vi "Peak Detection.vi"(7 "error in (no error)":errorcluster, 10 "Graph Data In":T1) -> (0 "error out":errorcluster, 2 "New Graph Data Out":T1)   [LabVIEW 2013, in "Diode Characterization.lvlib" / "Diode IV.lvclass"]
doc: "Detects up to 10 peaks per waveform that are above the threshold determined by the cursor on the graph. Output is in the form of an array of annotations that can be displayed on the graph alongside the input waveforms."
uses:
  Diode IV.lvclass
  graphdata.ctl
  <vilib>/Utility/miscctls.llb/LVAnnotationListTypeDef.ctl
  <vilib>/Utility/miscctls.llb/LVCursorListTypeDef.ctl
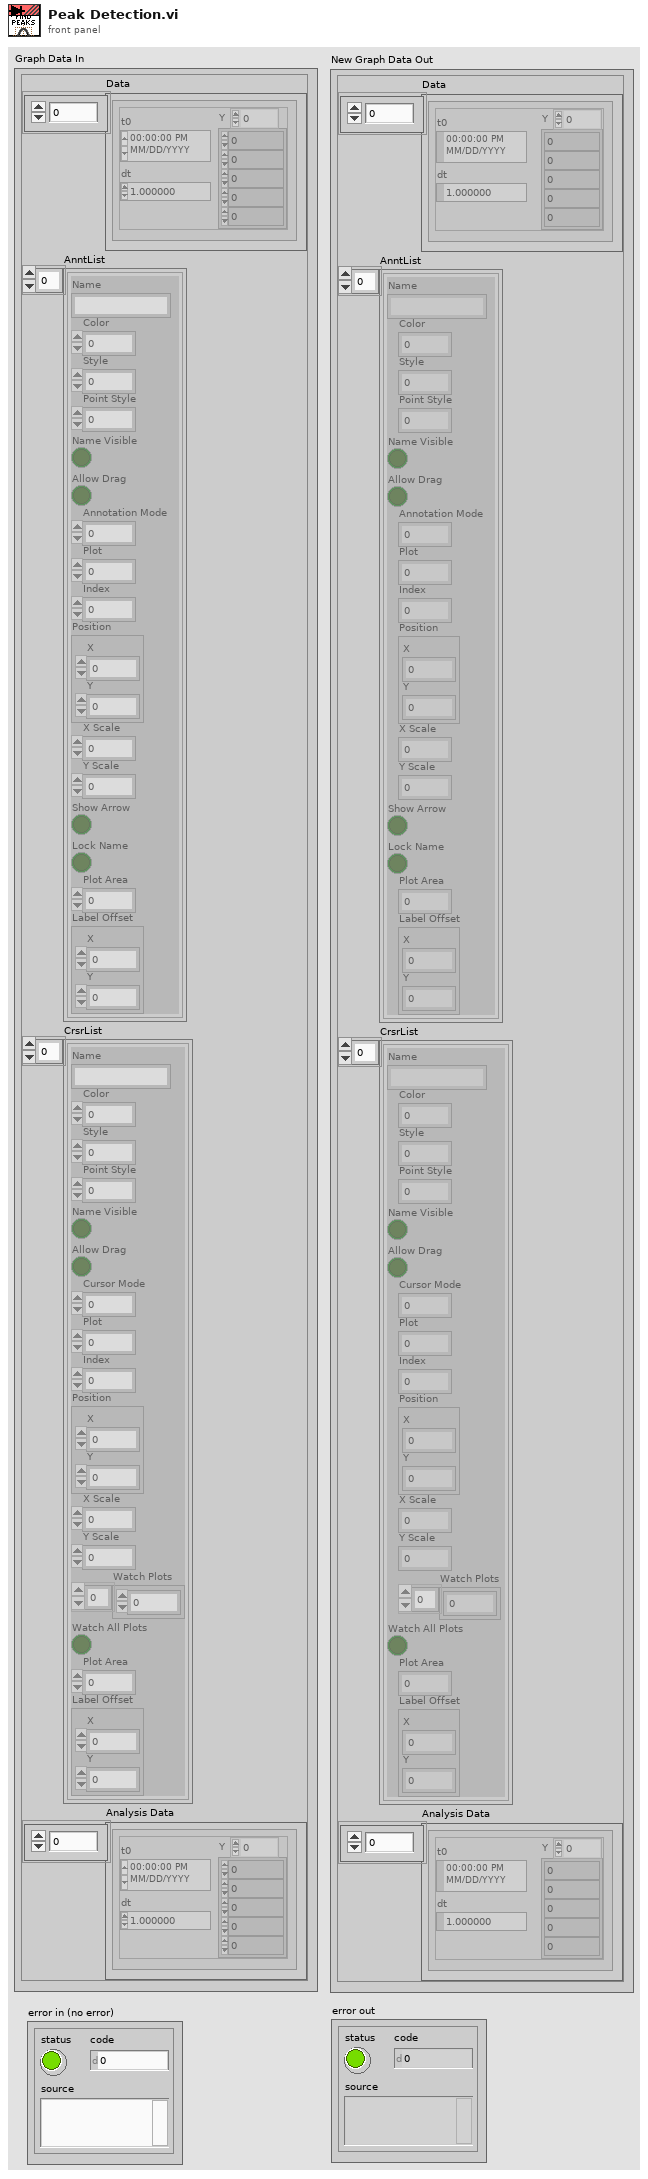
[diagram p1: front panel]
types:
  T1 = typedef "Diode Characterization.lvlib/Diode IV.lvclass/graphdata.ctl" = cluster{"Data":waveform(dbl)[], "AnntList":T2, "CrsrList":T3, "Analysis Data":waveform(dbl)[]}
  T2 = typedef "LVAnnotationListTypeDef.ctl" = cluster{"Name":string, "Color":u32, "Style":u8, "Point Style":u8, "Name Visible":bool, "Allow Drag":bool, "Annotation Mode":u32, "Plot":i32, "Index":i32, "Position":cluster{"X":dbl, "Y":dbl}, "X Scale":u32, "Y Scale":u32, "Show Arrow":bool, "Lock Name":bool, "Plot Area":i32, "Label Offset":cluster{"X":dbl, "Y":dbl}}[]
  T3 = typedef "LVCursorListTypeDef.ctl" = cluster{"Name":string, "Color":u32, "Style":u8, "Point Style":u8, "Name Visible":bool, "Allow Drag":bool, "Cursor Mode":u32, "Plot":i32, "Index":i32, "Position":cluster{"X":dbl, "Y":dbl}, "X Scale":u32, "Y Scale":u32, "Watch Plots":i32[], "Watch All Plots":bool, "Plot Area":i32, "Label Offset":cluster{"X":dbl, "Y":dbl}}[]
  T4 = cluster{"Name":string, "Color":u32, "Style":u8, "Point Style":u8, "Name Visible":bool, "Allow Drag":bool, "Cursor Mode":u32, "Plot":i32, "Index":i32, "Position":cluster{"X":dbl, "Y":dbl}, "X Scale":u32, "Y Scale":u32, "Watch Plots":i32[], "Watch All Plots":bool, "Plot Area":i32, "Label Offset":cluster{"X":dbl, "Y":dbl}}
  T5 = cluster{"Name":string, "Color":u32, "Style":u8, "Point Style":u8, "Name Visible":bool, "Allow Drag":bool, "Annotation Mode":u32, "Plot":i32, "Index":i32, "Position":cluster{"X":dbl, "Y":dbl}, "X Scale":u32, "Y Scale":u32, "Show Arrow":bool, "Lock Name":bool, "Plot Area":i32, "Label Offset":cluster{"X":dbl, "Y":dbl}}[]
  T6 = cluster{"Name":string, "Color":u32, "Style":u8, "Point Style":u8, "Name Visible":bool, "Allow Drag":bool, "Annotation Mode":u32, "Plot":i32, "Index":i32, "Position":cluster{"X":dbl, "Y":dbl}, "X Scale":u32, "Y Scale":u32, "Show Arrow":bool, "Lock Name":bool, "Plot Area":i32, "Label Offset":cluster{"X":dbl, "Y":dbl}}
  T7 = cluster{"Name":string, "Color":u32, "Style":u8, "Point Style":u8, "Name Visible":bool, "Allow Drag":bool, "Cursor Mode":u32, "Plot":i32, "Index":i32, "Position":cluster{"X":dbl, "Y":dbl}, "X Scale":u32, "Y Scale":u32, "Watch Plots":i32[], "Watch All Plots":bool, "Plot Area":i32, "Label Offset":cluster{"X":dbl, "Y":dbl}}[]
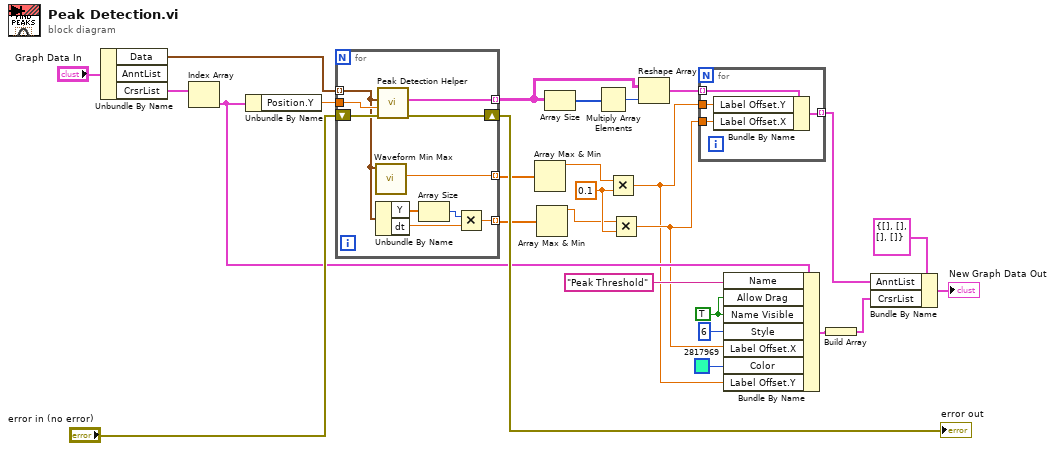
[diagram p0: block diagram]
diagram:
  w6 = 0.1 ("y")
  w14 = TRUE ("Allow Drag")
  n1 = Unbundle By Name("Graph Data In") -> ("Data"=w23:waveform(dbl)[], "CrsrList"=w24:T3)  [unwired: 1 out]
  n2 = Index Array(array=w24) -> (element=w17:T4)  [unwired: 1 in]
  n3 = Unbundle By Name(w17) -> ("Position.Y"=w18:dbl)
  n4 = for {
    tunnel: w23 -> [w29] mode=indexing
    tunnel: [w37] -> w21 mode=indexing
    tunnel: w18 -> [w36]
    shift-right: [w34] -> w27
    shift-left: "error in (no error)" -> [w35]
    tunnel: [w33] -> w9 mode=indexing
    tunnel: [w28] -> w8 mode=indexing
    n5 = call <vilib>:"Waveform Min Max.vi"("waveform in"=w29) -> ("Y max"=w33:dbl)  [unwired: 5 in, 5 out]
    n6 = Unbundle By Name(w29) -> ("Y"=w30:dbl[], "dt"=w32:dbl)
    n7 = call "Peak Detection Helper.vi"("Error In"=w35, "threshold"=w36, "Waveform"=w29) -> ("Error Out"=w34:errorcluster, "Annotations"=w37:T5)  [unwired: 7 in]
    n8 = Array Size(array=w30) -> (size(s)=w31:i32)
    n9 = Multiply(x=w31, y=w32) -> (x*y=w28:dbl)
  }
  "error out" <- w27
  n10 = Array Max & Min(array=w9) -> (max value=w3:dbl)  [unwired: 3 out]
  n11 = Array Max & Min(array=w8) -> (max value=w4:dbl)  [unwired: 3 out]
  n12 = Array Size(array=w21) -> (size(s)=w20:i32[])
  n13 = Multiply Array Elements(1:w20) -> (0:w19:i32)
  n14 = Multiply(x=w3, y=w6) -> (x*y=w1:dbl)
  n15 = Multiply(x=w4, y=w6) -> (x*y=w2:dbl)
  n16 = Reshape Array(w21, w19) -> (w7:T5)
  n17 = for {
    tunnel: w7 -> [w41] mode=indexing
    tunnel: w1 -> [w40]
    tunnel: w2 -> [w39]
    tunnel: [w38] -> w5 mode=indexing
    n18 = Bundle By Name(cluster=w41, "Label Offset.Y"=w40, "Label Offset.X"=w39) -> (w38:T6)
  }
  n19 = Bundle By Name(cluster=w17, "Name"="Peak Threshold", "Allow Drag"=w14, "Name Visible"=w14, "Style"=u8 6, "Label Offset.X"=w2, "Color"=u32 2817969, "Label Offset.Y"=w1) -> (w13:T4)
  n20 = Build Array(w13) -> (w25:T7)
  n21 = Bundle By Name(cluster=T1 {"Data"=[], "AnntList"=[], "CrsrList"=[], "Analysis Data"=[]} ("Graph Data In"), "AnntList"=w5, "CrsrList"=w25) -> (→"New Graph Data Out":T1)
